vi "REPORT.Rate scan.vi"(9 "Vasic":i32, 10 "Config Test IN":T1={"Config HW"={"VISA Rigol DP832"="USB0::0x1AB1::0x0E11::DP8C191500901::INSTR", "Config Rigol DP832"=[{"Channel"=0, "V Limit"=5.5, "I Limit"=0.5, "V Out"=5.0}, {"Channel"=1, "V Limit"=5.5, "I Limit"=0.8, "V Out"=5.0}, {"Channel"=2, "V Limit"=5.5, "I Limit"=0.2, "V Out"=0.0}], "CTA Test#"="CTA013 A", "FT_Handle"=432866568, "Espera acceso FT"=10, "VISA Tek MDO3104"="Rigol_DP832", "VISA Key 81160A"="Rigol_DP832"}, "Config Test"=[{"Vasic"=2.8, "Global Reset"=FALSE, "Test Register?"=FALSE, "Test ADC?"=FALSE, "Test ADC"={"Repeats ADC"=100, "Max Desviation"=0.1}, "Limits ADC"={"Low"=[1.9, 1.3, 0.65, 0.0, 1.6, 1.4, 1.4, 0.9, 2.1, 0.85, 1.9], "High"=[2.1, 1.5, 0.85, 0.1, 1.4, 1.2, 1.2, 0.7, 1.9, 0.65, 1.7]}, "Test Max PN Min NP?"=FALSE, "Limits Max PN Min NP"={"Max P Upper"=2.177000045776367, "Min P Upper"=1.474, "Max N Upper"=1.475, "Min N Upper"=0.818, "Max P Lower"=1.888, "Min P Lower "=1.321, "Max N Lower"=1.322, "Min N Lower"=0.73}, "Test Rate Scan?"=FALSE, "Vin Rate Scan"=[], "Limits Rate Scan"={"High"=[0.15, 0.242, 0.331, 0.425, 0.512, 0.6, 0.688, 0.774, 0.847, 0.91], "Low"=[0.021, 0.11, 0.189, 0.27, 0.347, 0.421, 0.487, 0.551, 0.601, 0.635]}, "Test Rate Scan Adders?"=FALSE, "Vin Rate Adders"=[], "Limits Rate Scan adders"={"High"=[], "Low"=[]}, "Test offset analog?"=FALSE, "Lim Offset Analog"={"Max Analog"=0.05, "Min Analog"=-0.05}, "Test offset digital?"=FALSE, "Lim offset Dig"={"Max Dig"=0.05}, "Vasic real f.a."=2.8, "IBIAS"=FALSE, "VALUE IBIAS"=63}, {"Vasic"=2.8, "Global Reset"=FALSE, "Test Register?"=FALSE, "Test ADC?"=FALSE, "Test ADC"={"Repeats ADC"=100, "Max Desviation"=0.1}, "Limits ADC"={"Low"=[1.9, 1.3, 0.65, 0.0, 1.6, 1.4, 1.4, 0.9, 2.1, 0.85, 1.9], "High"=[2.1, 1.5, 0.85, 0.1, 1.4, 1.2, 1.2, 0.7, 1.9, 0.65, 1.7]}, "Test Max PN Min NP?"=FALSE, "Limits Max PN Min NP"={"Max P Upper"=2.177000045776367, "Min P Upper"=1.474, "Max N Upper"=1.475, "Min N Upper"=0.818, "Max P Lower"=1.888, "Min P Lower "=1.321, "Max N Lower"=1.322, "Min N Lower"=0.73}, "Test Rate Scan?"=FALSE, "Vin Rate Scan"=[], "Limits Rate Scan"={"High"=[0.15, 0.242, 0.331, 0.425, 0.512, 0.6, 0.688, 0.774, 0.847, 0.91], "Low"=[0.021, 0.11, 0.189, 0.27, 0.347, 0.421, 0.487, 0.551, 0.601, 0.635]}, "Test Rate Scan Adders?"=FALSE, "Vin Rate Adders"=[], "Limits Rate Scan adders"={"High"=[], "Low"=[]}, "Test offset analog?"=FALSE, "Lim Offset Analog"={"Max Analog"=0.05, "Min Analog"=-0.05}, "Test offset digital?"=FALSE, "Lim offset Dig"={"Max Dig"=0.05}, "Vasic real f.a."=2.8, "IBIAS"=FALSE, "VALUE IBIAS"=63}, {"Vasic"=2.8, "Global Reset"=FALSE, "Test Register?"=FALSE, "Test ADC?"=FALSE, "Test ADC"={"Repeats ADC"=100, "Max Desviation"=0.1}, "Limits ADC"={"Low"=[1.9, 1.3, 0.65, 0.0, 1.6, 1.4, 1.4, 0.9, 2.1, 0.85, 1.9], "High"=[2.1, 1.5, 0.85, 0.1, 1.4, 1.2, 1.2, 0.7, 1.9, 0.65, 1.7]}, "Test Max PN Min NP?"=FALSE, "Limits Max PN Min NP"={"Max P Upper"=2.177000045776367, "Min P Upper"=1.474, "Max N Upper"=1.475, "Min N Upper"=0.818, "Max P Lower"=1.888, "Min P Lower "=1.321, "Max N Lower"=1.322, "Min N Lower"=0.73}, "Test Rate Scan?"=FALSE, "Vin Rate Scan"=[], "Limits Rate Scan"={"High"=[0.15, 0.242, 0.331, 0.425, 0.512, 0.6, 0.688, 0.774, 0.847, 0.91], "Low"=[0.021, 0.11, 0.189, 0.27, 0.347, 0.421, 0.487, 0.551, 0.601, 0.635]}, "Test Rate Scan Adders?"=FALSE, "Vin Rate Adders"=[], "Limits Rate Scan adders"={"High"=[], "Low"=[]}, "Test offset analog?"=FALSE, "Lim Offset Analog"={"Max Analog"=0.05, "Min Analog"=-0.05}, "Test offset digital?"=FALSE, "Lim offset Dig"={"Max Dig"=0.05}, "Vasic real f.a."=2.8, "IBIAS"=FALSE, "VALUE IBIAS"=63}, {"Vasic"=2.8, "Global Reset"=FALSE, "Test Register?"=FALSE, "Test ADC?"=FALSE, "Test ADC"={"Repeats ADC"=100, "Max Desviation"=0.1}, "Limits ADC"={"Low"=[1.9, 1.3, 0.65, 0.0, 1.6, 1.4, 1.4, 0.9, 2.1, 0.85, 1.9], "High"=[2.1, 1.5, 0.85, 0.1, 1.4, 1.2, 1.2, 0.7, 1.9, 0.65, 1.7]}, "Test Max PN Min NP?"=FALSE, "Limits Max PN Min NP"={"Max P Upper"=2.177000045776367, "Min P Upper"=1.474, "Max N Upper"=1.475, "Min N Upper"=0.818, "Max P Lower"=1.888, "Min P Lower "=1.321, "Max N Lower"=1.322, "Min N Lower"=0.73}, "Test Rate Scan?"=FALSE, "Vin Rate Scan"=[], "Limits Rate Scan"={"High"=[0.15, 0.242, 0.331, 0.425, 0.512, 0.6, 0.688, 0.774, 0.847, 0.91], "Low"=[0.021, 0.11, 0.189, 0.27, 0.347, 0.421, 0.487, 0.551, 0.601, 0.635]}, "Test Rate Scan Adders?"=FALSE, "Vin Rate Adders"=[], "Limits Rate Scan adders"={"High"=[], "Low"=[]}, "Test offset analog?"=FALSE, "Lim Offset Analog"={"Max Analog"=0.05, "Min Analog"=-0.05}, "Test offset digital?"=FALSE, "Lim offset Dig"={"Max Dig"=0.05}, "Vasic real f.a."=2.8, "IBIAS"=FALSE, "VALUE IBIAS"=63}], "Result"=[{"Vasic Volt"=0, "Test Registros"={"Default Register OK"=FALSE, "Pattern Default"=[], "Read Default"=[], "W/R Register OK"=FALSE, "Pattern W/R"=[], "Read W/R"=[]}, "Test Dacs"={"Desviacion OK"=FALSE, "Means"=[], "Deviations"=[], "Desviations OK"=[], "Means OK"=[], "Graph Histogram"=[]}, "Test Max-Min PN"={"Max P Mini N OK"=FALSE, "PTHT Max P Min N"=[], "PTHT Max P Min N OK"=[], "NTHT Max P Min N"=[], "NTHT Max P Min N OK"=[], "Min P Max N OK"=FALSE, "PTHT Max N Min P"=[], "PTHT Max N Min P OK"=[], "NTHT Max N Min P"=[], "NTHT Max N Min P OK"=[], "Ref"=[]}, "Test Rate Scan"={"Rate Scan OK"=FALSE, "DAC TH0,TH1,TH2"=[], "Volt HLTH"=[], "Rate HLTH OK"=[], "DAC TH3,TH4,TH5"=[], "Volt LLTH"=[], "Rate LLTH 2 OK"=[], "Scaler 0"=[], "Ref"=[], "OFFSET HLTH"=[], "OFFSET LLTH"=[], "Real Voltage"=[]}, "Test Rate Scan adders"={"Rate Scan Adders OK"=FALSE, "DAC TH0,TH1,TH2"=[], "Volt HLTH"=[], "Add HLTH OK"=[], "DAC TH3,TH4,TH5"=[], "Volt LLTH"=[], "Add LLTH 2 OK"=[], "Scaler 0"=[], "Ref"=[], "OFFSET HLTH"=[], "OFFSET LLTH"=[], "Real Voltage"=[]}, "Test Offset Analog"={"Offset Analog OK"=FALSE, "V ADDOUT"=[], "Offset OK"=[], "Ref"=[]}, "Test Offset Digital"={"Offset Digital OK"=FALSE, "SCALER 1 START"=[], "SCALER 1 STOP"=[], "THX START"=[], "THX STOP"=[], "VHLTH START"=[], "VHLTH STOP"=[], "Index 1 Start"=[], "index 1 Stop"=[], "SCALER 2 START"=[], "SCALER 2 STOP"=[], "THX+3 START"=[], "THX+3 STOP"=[], "VLLTH START"=[], "VLLTH STOP"=[], "Index 2 Start"=[], "index 2 Stop"=[], "Dig HLTH OK"=[], "Dig LLTH 2 OK"=[], "Ref"=[]}, "info hardware"={"Iout V1"=0.0, "Iout V2"=0.0, "Iout V3"=0.0, "Vout V1"=0.0, "Vout V2"=0.0, "Vout V3"=0.0, "Temp"=0.0}, "Test Offset Analog add"={"Offset Analog add OK"=FALSE, "V ADDOUT add"=[], "Offset add OK"=[], "Ref add"=[]}, "info temp"={"T Asic Registers"=0.0, "T Board Test. ADC"=0.0, "T Asic Max Min N P"=0.0, "T Adc count"=0.0, "T Asic Digital Offset"=0.0, "T Asic Analog Offset"=0.0, "T Asic Analog add"=0.0, "T Asic Rate Scan"=0.0, "T Asic Rate Scan Adders"=0.0, "T Final"=0.0}}, {"Vasic Volt"=0, "Test Registros"={"Default Register OK"=FALSE, "Pattern Default"=[], "Read Default"=[], "W/R Register OK"=FALSE, "Pattern W/R"=[], "Read W/R"=[]}, "Test Dacs"={"Desviacion OK"=FALSE, "Means"=[], "Deviations"=[], "Desviations OK"=[], "Means OK"=[], "Graph Histogram"=[]}, "Test Max-Min PN"={"Max P Mini N OK"=FALSE, "PTHT Max P Min N"=[], "PTHT Max P Min N OK"=[], "NTHT Max P Min N"=[], "NTHT Max P Min N OK"=[], "Min P Max N OK"=FALSE, "PTHT Max N Min P"=[], "PTHT Max N Min P OK"=[], "NTHT Max N Min P"=[], "NTHT Max N Min P OK"=[], "Ref"=[]}, "Test Rate Scan"={"Rate Scan OK"=FALSE, "DAC TH0,TH1,TH2"=[], "Volt HLTH"=[], "Rate HLTH OK"=[], "DAC TH3,TH4,TH5"=[], "Volt LLTH"=[], "Rate LLTH 2 OK"=[], "Scaler 0"=[], "Ref"=[], "OFFSET HLTH"=[], "OFFSET LLTH"=[], "Real Voltage"=[]}, "Test Rate Scan adders"={"Rate Scan Adders OK"=FALSE, "DAC TH0,TH1,TH2"=[], "Volt HLTH"=[], "Add HLTH OK"=[], "DAC TH3,TH4,TH5"=[], "Volt LLTH"=[], "Add LLTH 2 OK"=[], "Scaler 0"=[], "Ref"=[], "OFFSET HLTH"=[], "OFFSET LLTH"=[], "Real Voltage"=[]}, "Test Offset Analog"={"Offset Analog OK"=FALSE, "V ADDOUT"=[], "Offset OK"=[], "Ref"=[]}, "Test Offset Digital"={"Offset Digital OK"=FALSE, "SCALER 1 START"=[], "SCALER 1 STOP"=[], "THX START"=[], "THX STOP"=[], "VHLTH START"=[], "VHLTH STOP"=[], "Index 1 Start"=[], "index 1 Stop"=[], "SCALER 2 START"=[], "SCALER 2 STOP"=[], "THX+3 START"=[], "THX+3 STOP"=[], "VLLTH START"=[], "VLLTH STOP"=[], "Index 2 Start"=[], "index 2 Stop"=[], "Dig HLTH OK"=[], "Dig LLTH 2 OK"=[], "Ref"=[]}, "info hardware"={"Iout V1"=0.0, "Iout V2"=0.0, "Iout V3"=0.0, "Vout V1"=0.0, "Vout V2"=0.0, "Vout V3"=0.0, "Temp"=0.0}, "Test Offset Analog add"={"Offset Analog add OK"=FALSE, "V ADDOUT add"=[], "Offset add OK"=[], "Ref add"=[]}, "info temp"={"T Asic Registers"=0.0, "T Board Test. ADC"=0.0, "T Asic Max Min N P"=0.0, "T Adc count"=0.0, "T Asic Digital Offset"=0.0, "T Asic Analog Offset"=0.0, "T Asic Analog add"=0.0, "T Asic Rate Scan"=0.0, "T Asic Rate Scan Adders"=0.0, "T Final"=0.0}}, {"Vasic Volt"=0, "Test Registros"={"Default Register OK"=FALSE, "Pattern Default"=[], "Read Default"=[], "W/R Register OK"=FALSE, "Pattern W/R"=[], "Read W/R"=[]}, "Test Dacs"={"Desviacion OK"=FALSE, "Means"=[], "Deviations"=[], "Desviations OK"=[], "Means OK"=[], "Graph Histogram"=[]}, "Test Max-Min PN"={"Max P Mini N OK"=FALSE, "PTHT Max P Min N"=[], "PTHT Max P Min N OK"=[], "NTHT Max P Min N"=[], "NTHT Max P Min N OK"=[], "Min P Max N OK"=FALSE, "PTHT Max N Min P"=[], "PTHT Max N Min P OK"=[], "NTHT Max N Min P"=[], "NTHT Max N Min P OK"=[], "Ref"=[]}, "Test Rate Scan"={"Rate Scan OK"=FALSE, "DAC TH0,TH1,TH2"=[], "Volt HLTH"=[], "Rate HLTH OK"=[], "DAC TH3,TH4,TH5"=[], "Volt LLTH"=[], "Rate LLTH 2 OK"=[], "Scaler 0"=[], "Ref"=[], "OFFSET HLTH"=[], "OFFSET LLTH"=[], "Real Voltage"=[]}, "Test Rate Scan adders"={"Rate Scan Adders OK"=FALSE, "DAC TH0,TH1,TH2"=[], "Volt HLTH"=[], "Add HLTH OK"=[], "DAC TH3,TH4,TH5"=[], "Volt LLTH"=[], "Add LLTH 2 OK"=[], "Scaler 0"=[], "Ref"=[], "OFFSET HLTH"=[], "OFFSET LLTH"=[], "Real Voltage"=[]}, "Test Offset Analog"={"Offset Analog OK"=FALSE, "V ADDOUT"=[], "Offset OK"=[], "Ref"=[]}, "Test Offset Digital"={"Offset Digital OK"=FALSE, "SCALER 1 START"=[], "SCALER 1 STOP"=[], "THX START"=[], "THX STOP"=[], "VHLTH START"=[], "VHLTH STOP"=[], "Index 1 Start"=[], "index 1 Stop"=[], "SCALER 2 START"=[], "SCALER 2 STOP"=[], "THX+3 START"=[], "THX+3 STOP"=[], "VLLTH START"=[], "VLLTH STOP"=[], "Index 2 Start"=[], "index 2 Stop"=[], "Dig HLTH OK"=[], "Dig LLTH 2 OK"=[], "Ref"=[]}, "info hardware"={"Iout V1"=0.0, "Iout V2"=0.0, "Iout V3"=0.0, "Vout V1"=0.0, "Vout V2"=0.0, "Vout V3"=0.0, "Temp"=0.0}, "Test Offset Analog add"={"Offset Analog add OK"=FALSE, "V ADDOUT add"=[], "Offset add OK"=[], "Ref add"=[]}, "info temp"={"T Asic Registers"=0.0, "T Board Test. ADC"=0.0, "T Asic Max Min N P"=0.0, "T Adc count"=0.0, "T Asic Digital Offset"=0.0, "T Asic Analog Offset"=0.0, "T Asic Analog add"=0.0, "T Asic Rate Scan"=0.0, "T Asic Rate Scan Adders"=0.0, "T Final"=0.0}}, {"Vasic Volt"=0, "Test Registros"={"Default Register OK"=FALSE, "Pattern Default"=[], "Read Default"=[], "W/R Register OK"=FALSE, "Pattern W/R"=[], "Read W/R"=[]}, "Test Dacs"={"Desviacion OK"=FALSE, "Means"=[], "Deviations"=[], "Desviations OK"=[], "Means OK"=[], "Graph Histogram"=[]}, "Test Max-Min PN"={"Max P Mini N OK"=FALSE, "PTHT Max P Min N"=[], "PTHT Max P Min N OK"=[], "NTHT Max P Min N"=[], "NTHT Max P Min N OK"=[], "Min P Max N OK"=FALSE, "PTHT Max N Min P"=[], "PTHT Max N Min P OK"=[], "NTHT Max N Min P"=[], "NTHT Max N Min P OK"=[], "Ref"=[]}, "Test Rate Scan"={"Rate Scan OK"=FALSE, "DAC TH0,TH1,TH2"=[], "Volt HLTH"=[], "Rate HLTH OK"=[], "DAC TH3,TH4,TH5"=[], "Volt LLTH"=[], "Rate LLTH 2 OK"=[], "Scaler 0"=[], "Ref"=[], "OFFSET HLTH"=[], "OFFSET LLTH"=[], "Real Voltage"=[]}, "Test Rate Scan adders"={"Rate Scan Adders OK"=FALSE, "DAC TH0,TH1,TH2"=[], "Volt HLTH"=[], "Add HLTH OK"=[], "DAC TH3,TH4,TH5"=[], "Volt LLTH"=[], "Add LLTH 2 OK"=[], "Scaler 0"=[], "Ref"=[], "OFFSET HLTH"=[], "OFFSET LLTH"=[], "Real Voltage"=[]}, "Test Offset Analog"={"Offset Analog OK"=FALSE, "V ADDOUT"=[], "Offset OK"=[], "Ref"=[]}, "Test Offset Digital"={"Offset Digital OK"=FALSE, "SCALER 1 START"=[], "SCALER 1 STOP"=[], "THX START"=[], "THX STOP"=[], "VHLTH START"=[], "VHLTH STOP"=[], "Index 1 Start"=[], "index 1 Stop"=[], "SCALER 2 START"=[], "SCALER 2 STOP"=[], "THX+3 START"=[], "THX+3 STOP"=[], "VLLTH START"=[], "VLLTH STOP"=[], "Index 2 Start"=[], "index 2 Stop"=[], "Dig HLTH OK"=[], "Dig LLTH 2 OK"=[], "Ref"=[]}, "info hardware"={"Iout V1"=0.0, "Iout V2"=0.0, "Iout V3"=0.0, "Vout V1"=0.0, "Vout V2"=0.0, "Vout V3"=0.0, "Temp"=0.0}, "Test Offset Analog add"={"Offset Analog add OK"=FALSE, "V ADDOUT add"=[], "Offset add OK"=[], "Ref add"=[]}, "info temp"={"T Asic Registers"=0.0, "T Board Test. ADC"=0.0, "T Asic Max Min N P"=0.0, "T Adc count"=0.0, "T Asic Digital Offset"=0.0, "T Asic Analog Offset"=0.0, "T Asic Analog add"=0.0, "T Asic Rate Scan"=0.0, "T Asic Rate Scan Adders"=0.0, "T Final"=0.0}}], "Execucion Test"={"Vasic Actual"=0}, "Config VGA"={"Theoretical Voltage"=[0.1, 0.2, 0.3, 0.4, 0.5, 0.6, 0.7, 0.8, 0.9, 1.0], "Real Voltage"=[0.10285, 0.20714, 0.29957, 0.40485, 0.49571, 0.60685, 0.69771, 0.80114, 0.89714, 0.99885], "Pulse Width"=57344, "Frecuency Pulse"=1000000.0, "VGA Gain"=[9, 16, 24, 34, 43, 52, 61, 72, 81, 93]}, "Test Info"={"Asic"="", "Operator"="", "Place"="", "Time start"=timestamp(0 s since 1904-01-01), "Time stop"=timestamp(0 s since 1904-01-01)}, "Info machine"={"SO"="", "SO Name"="", "SO Ver"="", "SO Build"="", "CPU"="", "APP"="", "APP YEAR"="", "APP ver"="", "APP User"="", "APP Serail"="", "MAC"=[], "PC NAME"=[], "PC IP"=[], "BIOS MANU"="", "BIOS NAME"="", "BIOS SERIAL"="", "BOARD MANU"="", "BOARD NAME"="", "BOARD SERIAL"="", "Driver Version"="", "Library Version"="", "FPGA Ver"=0, "ID CTA board"=0, "LAST BOOT"="", "LABVIEW Ver"=0}, "Partial Report"="", "CONFIG GEN"=[]} {"CONFIG GEN"."Vasic Theorical" min=1.0 max=1000000.0 step=1.0 format="%#_6pV"; "CONFIG GEN"."Frequency" min=0.001 max=333000000.0 step=1000.0 format="%#_6pHz"; "CONFIG GEN"."Leading Edge Time" min=1e-09 max=1.0 step=1e-10 format="%#_6ps"; "CONFIG GEN"."Trailing Edge Time" min=1e-09 max=1.0 step=1e-10 format="%#_6ps"; "CONFIG GEN"."Delay" min=0.0 max=1.0 step=1e-12 format="%#_6ps"; "CONFIG GEN"."Trigger Level Sync" items=["ECL", "TTL"]; "CONFIG GEN"."Trigger Sync Out" items=["AB"=3, "B"=2, "A"=1, "None"=0]; "CONFIG GEN"."Load" min=1.0 max=1000000.0 step=1.0 format="%#_6p"; "CONFIG GEN"."DC Offset" min=-10.0 max=10.0 step=0.1 format="%#_6pV"; "CONFIG GEN"."Amplitude" min=0.05 max=5.0 step=0.001 format="%#_6pV"; "CONFIG GEN"."Width Time" min=1.5e-09 max=1.0 step=1e-10 format="%#_6ps"; "CONFIG GEN"."Channel" items=["Channel1"=1, "Channel2"=2]; "Config VGA"."Theoretical Voltage" format="%1.4f"; "Config VGA"."VGA Gain" format="%02x"; "Config VGA"."Frecuency Pulse" format="%0_2p"; "Config VGA"."Pulse Width" format="%04x"; "Config VGA"."Real Voltage" format="%1.5f"; "Config Test"."VALUE IBIAS" max=63 step=1; "Config Test"."Vasic real f.a." min=2.8 max=3.8 step=0.01 format="%.2g"; "Config Test"."Limits Rate Scan adders"."Low" format="%1.3f"; "Config Test"."Limits Rate Scan adders"."High" format="%1.3f"; "Config Test"."Limits ADC"."High" format="%1.4f"; "Config Test"."Limits ADC"."Low" format="%1.3f"; "Config Test"."Lim offset Dig"."Max Dig" format="%.3g"; "Config Test"."Lim Offset Analog"."Min Analog" format="%.3g"; "Config Test"."Lim Offset Analog"."Max Analog" format="%.3g"; "Config Test"."Limits Rate Scan"."Low" format="%1.4f"; "Config Test"."Limits Rate Scan"."High" format="%1.3f"; "Config Test"."Limits Max PN Min NP"."Min P Upper" format="%.3g"; "Config Test"."Limits Max PN Min NP"."Min P Lower" format="%.3g"; "Config Test"."Limits Max PN Min NP"."Max N Lower" format="%.3g"; "Config Test"."Limits Max PN Min NP"."Max N Upper" format="%.3g"; "Config Test"."Limits Max PN Min NP"."Min N Lower" format="%.3g"; "Config Test"."Limits Max PN Min NP"."Min N Upper" format="%.3g"; "Config Test"."Limits Max PN Min NP"."Max P Upper" format="%.3g"; "Config Test"."Limits Max PN Min NP"."Max P Lower" format="%.3g"; "Config Test"."Vasic" min=2.8 max=3.8 step=0.01 format="%.2g"; "Config HW"."Config Rigol DP832"."Channel" items=["+30V Channel 1", "+30V Channel 2", "+5V Channel 3"]; "Config HW"."Config Rigol DP832"."V Limit" format="%.1g"; "Config HW"."Config Rigol DP832"."I Limit" format="%.1g"; "Config HW"."Config Rigol DP832"."V Out" format="%.1g"; "Result"."Test Registros"."Read W/R" format="%04x"; "Result"."Test Registros"."Pattern W/R" format="%04x"; "Result"."Test Registros"."Read Default" format="%04x"; "Result"."Test Registros"."Pattern Default" format="%04x"}, 11 "Text In":string) -> (3 "Text Out":string)   [LabVIEW 2019]
uses:
  Test.ctl
  TEST.TEST CONFIG HW.ctl
  Rigol DP832/DP832_Control Channels.ctl
  TEST.TEST CONFIG TEST MATRIZ.ctl
  TEST.TEST CONFIG TEST.ctl
  TEST.TEST RESULT.ctl
  test_result fvasic.ctl
  TEST.TEST EXECUTION TEST.ctl
  TEST.TEST CONFIG VGA.ctl
  TEST.TEST TEST INFO.ctl
  TEST.TEST INFO PC.ctl
  GenPulse_configurar.ctl
panel:
  out "Test Rate Scan.OFFSET LLTH":dbl[][](array[numeric])
  out "Test Rate Scan.OFFSET HLTH":dbl[][](array[numeric])
  out "Salida B rectificada":dbl[][][](array[numeric])
  out "Salida A rectificada":dbl[][][](array[numeric])
  # "Modo 2\nModo 3\nModo 4\nModo 2\nModo 3\nModo 4"
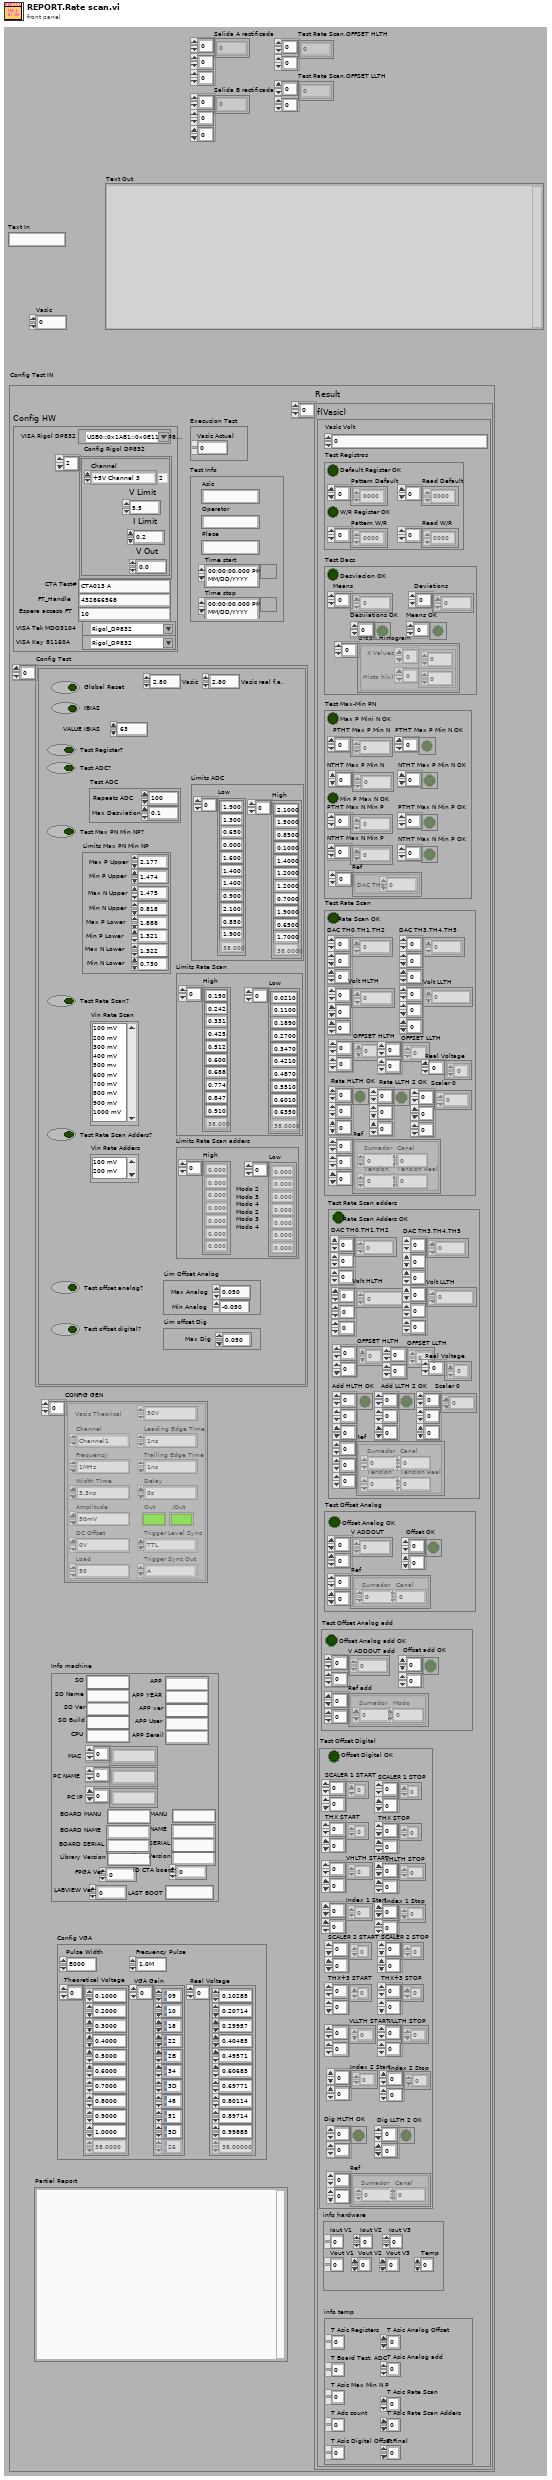
[diagram p1: front panel]
types:
  T1 = typedef "Test.ctl" = cluster{"Config HW":T2, "Config Test":T4, "Result":T6, "Execucion Test":T8, "Config VGA":T9, "Test Info":T10, "Info machine":T11, "Partial Report":string, "CONFIG GEN":T12[]}
  T2 = typedef "TEST.TEST CONFIG HW.ctl" = cluster{"VISA Rigol DP832":refnum<visa-resource-name>, "Config Rigol DP832":cluster{"Channel":T3, "V Limit":dbl, "I Limit":dbl, "V Out":dbl}[], "CTA Test#":string, "FT_Handle":u32, "Espera acceso FT":u32, "VISA Tek MDO3104":refnum<visa-resource-name>, "VISA Key 81160A":refnum<visa-resource-name>}
  T3 = typedef "DP832_Control Channels.ctl" = i32
  T4 = typedef "TEST.TEST CONFIG TEST MATRIZ.ctl" = T5[]
  T5 = typedef "TEST.TEST CONFIG TEST.ctl" = cluster{"Vasic":dbl, "Global Reset":bool, "Test Register?":bool, "Test ADC?":bool, "Test ADC":cluster{"Repeats ADC":i32, "Max Desviation":dbl}, "Limits ADC":cluster{"Low":dbl[], "High":dbl[]}, "Test Max PN Min NP?":bool, "Limits Max PN Min NP":cluster{"Max P Upper":dbl, "Min P Upper":dbl, "Max N Upper":dbl, "Min N Upper":dbl, "Max P Lower":dbl, "Min P Lower ":dbl, "Max N Lower":dbl, "Min N Lower":dbl}, "Test Rate Scan?":bool, "Vin Rate Scan":i32[], "Limits Rate Scan":cluster{"High":dbl[], "Low":dbl[]}, "Test Rate Scan Adders?":bool, "Vin Rate Adders":i32[], "Limits Rate Scan adders":cluster{"High":dbl[], "Low":dbl[]}, "Test offset analog?":bool, "Lim Offset Analog":cluster{"Max Analog":dbl, "Min Analog":dbl}, "Test offset digital?":bool, "Lim offset Dig":cluster{"Max Dig":dbl}, "Vasic real f.a.":dbl, "IBIAS":bool, "VALUE IBIAS":u8}
  T6 = typedef "TEST.TEST RESULT.ctl" = T7[]
  T7 = typedef "test_result fvasic.ctl" = cluster{"Vasic Volt":i32, "Test Registros":cluster{"Default Register OK":bool, "Pattern Default":u16[], "Read Default":u16[], "W/R Register OK":bool, "Pattern W/R":u16[], "Read W/R":u16[]}, "Test Dacs":cluster{"Desviacion OK":bool, "Means":dbl[], "Deviations":dbl[], "Desviations OK":bool[], "Means OK":bool[], "Graph Histogram":cluster{"X Values":dbl[], "Histo h(x)":i32[]}[]}, "Test Max-Min PN":cluster{"Max P Mini N OK":bool, "PTHT Max P Min N":dbl[], "PTHT Max P Min N OK":bool[], "NTHT Max P Min N":dbl[], "NTHT Max P Min N OK":bool[], "Min P Max N OK":bool, "PTHT Max N Min P":dbl[], "PTHT Max N Min P OK":bool[], "NTHT Max N Min P":dbl[], "NTHT Max N Min P OK":bool[], "Ref":cluster{"DAC THx":u8}[]}, "Test Rate Scan":cluster{"Rate Scan OK":bool, "DAC TH0,TH1,TH2":u16[][][], "Volt HLTH":dbl[][][], "Rate HLTH OK":bool[][][], "DAC TH3,TH4,TH5":u16[][][], "Volt LLTH":dbl[][][], "Rate LLTH 2 OK":bool[][][], "Scaler 0":u16[][][], "Ref":cluster{"Sumador":u8, "Canal":u8, "Tension":u8, "Tension Real":dbl}[][][], "OFFSET HLTH":dbl[][], "OFFSET LLTH":dbl[][], "Real Voltage":dbl[]}, "Test Rate Scan adders":cluster{"Rate Scan Adders OK":bool, "DAC TH0,TH1,TH2":u16[][][], "Volt HLTH":dbl[][][], "Add HLTH OK":bool[][][], "DAC TH3,TH4,TH5":u16[][][], "Volt LLTH":dbl[][][], "Add LLTH 2 OK":bool[][][], "Scaler 0":u16[][][], "Ref":cluster{"Sumador":u8, "Canal":u8, "Tension":u8, "Tension Real":dbl}[][][], "OFFSET HLTH":dbl[][], "OFFSET LLTH":dbl[][], "Real Voltage":dbl[]}, "Test Offset Analog":cluster{"Offset Analog OK":bool, "V ADDOUT":dbl[][], "Offset OK":bool[][], "Ref":cluster{"Sumador":u8, "Canal":u8}[][]}, "Test Offset Digital":cluster{"Offset Digital OK":bool, "SCALER 1 START":u16[][], "SCALER 1 STOP":u16[][], "THX START":u16[][], "THX STOP":u16[][], "VHLTH START":dbl[][], "VHLTH STOP":dbl[][], "Index 1 Start":i32[][], "index 1 Stop":i32[][], "SCALER 2 START":u16[][], "SCALER 2 STOP":u16[][], "THX+3 START":u16[][], "THX+3 STOP":u16[][], "VLLTH START":dbl[][], "VLLTH STOP":dbl[][], "Index 2 Start":i32[][], "index 2 Stop":i32[][], "Dig HLTH OK":bool[][], "Dig LLTH 2 OK":bool[][], "Ref":cluster{"Sumador":u8, "Canal":u8}[][]}, "info hardware":cluster{"Iout V1":dbl, "Iout V2":dbl, "Iout V3":dbl, "Vout V1":dbl, "Vout V2":dbl, "Vout V3":dbl, "Temp":dbl}, "Test Offset Analog add":cluster{"Offset Analog add OK":bool, "V ADDOUT add":dbl[][], "Offset add OK":bool[][], "Ref add":cluster{"Sumador":u8, "Modo":u8}[][]}, "info temp":cluster{"T Asic Registers":dbl, "T Board Test. ADC":dbl, "T Asic Max Min N P":dbl, "T Adc count":dbl, "T Asic Digital Offset":dbl, "T Asic Analog Offset":dbl, "T Asic Analog add":dbl, "T Asic Rate Scan":dbl, "T Asic Rate Scan Adders":dbl, "T Final":dbl}}
  T8 = typedef "TEST.TEST EXECUTION TEST.ctl" = cluster{"Vasic Actual":i32}
  T9 = typedef "TEST.TEST CONFIG VGA.ctl" = cluster{"Theoretical Voltage":dbl[], "Real Voltage":dbl[], "Pulse Width":u16, "Frecuency Pulse":dbl, "VGA Gain":u8[]}
  T10 = typedef "TEST.TEST TEST INFO.ctl" = cluster{"Asic":string, "Operator":string, "Place":string, "Time start":timestamp, "Time stop":timestamp}
  T11 = typedef "TEST.TEST INFO PC.ctl" = cluster{"SO":string, "SO Name":string, "SO Ver":string, "SO Build":string, "CPU":string, "APP":string, "APP YEAR":string, "APP ver":string, "APP User":string, "APP Serail":string, "MAC":string[], "PC NAME":string[], "PC IP":string[], "BIOS MANU":string, "BIOS NAME":string, "BIOS SERIAL":string, "BOARD MANU":string, "BOARD NAME":string, "BOARD SERIAL":string, "Driver Version":string, "Library Version":string, "FPGA Ver":u8, "ID CTA board":u64, "LAST BOOT":string, "LABVIEW Ver":u32}
  T12 = typedef "GenPulse_configurar.ctl" = cluster{"Channel":u16, "Frequency":dbl, "Width Time":dbl, "Amplitude":dbl, "DC Offset":dbl, "Load":dbl, "Leading Edge Time":dbl, "Trailing Edge Time":dbl, "Delay":dbl, "Out":bool, "/Out":bool, "Trigger Level Sync":u16, "Trigger Sync Out":u16, "Vasic Theorical":dbl}
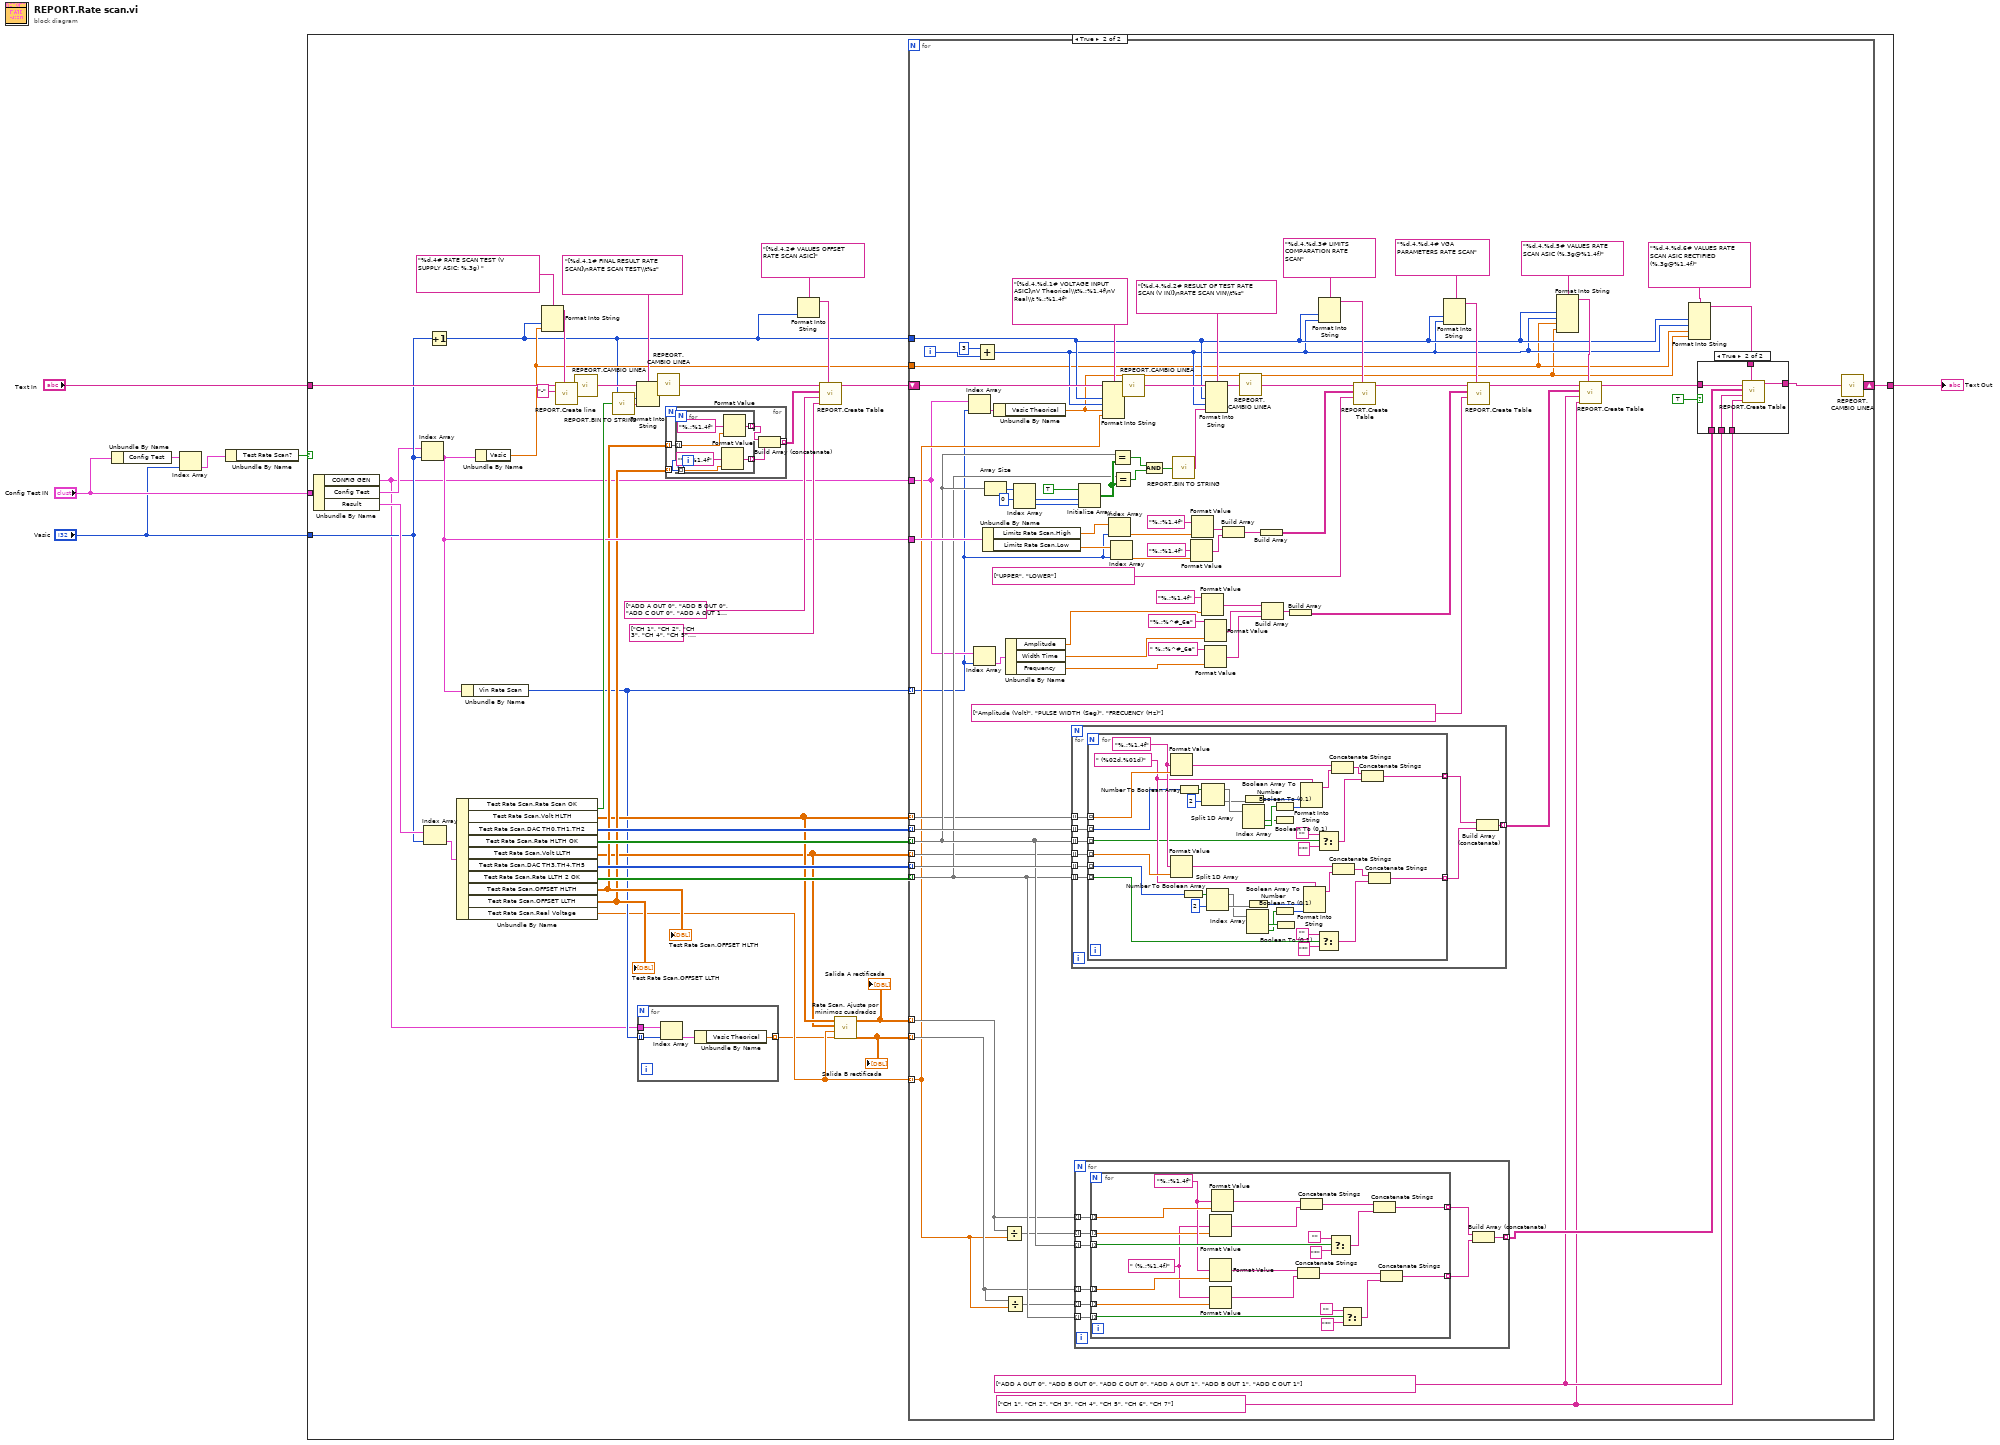
[diagram p0: block diagram]
diagram:
  n1 = Unbundle By Name("Config Test IN") -> ("Config Test"=w5:T4)
  n2 = Index Array(array=w5, index="Vasic") -> (element=w4:T5)
  n3 = Unbundle By Name(w4) -> ("Test Rate Scan?"=w2:bool)
  n4 = case shown="True" w2 {
    tunnel: "Text In" -> [w8 w48]
    tunnel: [w8 w44] -> w6
    tunnel: "Vasic" -> [_ w37]
    tunnel: "Config Test IN" -> [_ w30]
    frame False {
    }
    frame True {
      n5 = Unbundle By Name(w30) -> ("CONFIG GEN"=w9:T12[], "Config Test"=w13:T4, "Result"=w42:T6)
      n6 = Index Array(array=w13, index=w37) -> (element=w21:T5)
      n7 = Index Array(array=w42, index=w37) -> (element=w47:T7)
      n8 = Increment(x=w37) -> (x+1=w24:i32)
      n9 = Unbundle By Name(w47) -> ("Test Rate Scan.Rate Scan OK"=w32:bool, "Test Rate Scan.Volt HLTH"=w17:dbl[][][], "Test Rate Scan.DAC TH0,TH1,TH2"=w46:u16[][][], "Test Rate Scan.Rate HLTH OK"=w41:bool[][][], "Test Rate Scan.Volt LLTH"=w16:dbl[][][], "Test Rate Scan.DAC TH3,TH4,TH5"=w45:u16[][][], "Test Rate Scan.Rate LLTH 2 OK"=w40:bool[][][], "Test Rate Scan.OFFSET HLTH"=w20:dbl[][], "Test Rate Scan.OFFSET LLTH"=w19:dbl[][], "Test Rate Scan.Real Voltage"=w11:dbl[])
      "Test Rate Scan.OFFSET HLTH" <- w20
      "Test Rate Scan.OFFSET LLTH" <- w19
      n10 = Unbundle By Name(w21) -> ("Vin Rate Scan"=w12:i32[])
      n11 = Unbundle By Name(w21) -> ("Vasic"=w25:dbl)
      n12 = Format Into String(format string="%d.4# RATE SCAN TEST (V SUPPLY ASIC: %.3g) " ("Secction"), w24, w25) -> (resulting string=w36:string)  [unwired: 2 in, 1 out]
      n13 = call "REPORT.Create line.vi"("Secction"=w36, "Char"="-", "Text In"=w48) -> ("Text Out"=w43:string)  [unwired: 8 in]
      n14 = call "REPEORT.CAMBIO LINEA.vi"("Text Out"=w43) -> ("String"=w34:string)  [unwired: 8 in]
      n15 = call "REPORT.BIN TO STRING.vi"("Resultado test"=w32) -> ("OK, Fault"=w33:string)  [unwired: 14 in]
      n16 = Format Into String(format string="[%d.4.1# FINAL RESULT RATE SCAN]\nRATE SCAN TEST\\t%s" ("Secction"), initial string=w34, w24, w33) -> (resulting string=w31:string)  [unwired: 1 in, 1 out]
      n17 = for {
        tunnel: w12 -> [w52] mode=indexing
        tunnel: w9 -> [w51]
        tunnel: [w49] -> w10 mode=indexing
        n18 = Index Array(array=w51, index=w52) -> (element=w50:T12)
        n19 = Unbundle By Name(w50) -> ("Vasic Theorical"=w49:dbl)
      }
      n20 = call "REPEORT.CAMBIO LINEA.vi"("Text Out"=w31) -> ("String"=w27:string)  [unwired: 8 in]
      n21 = for {
        tunnel: w20 -> [w57] mode=indexing
        tunnel: w19 -> [w56] mode=indexing
        tunnel: [w53] -> w18 mode=indexing
        n22 = for {
          tunnel: w57 -> [w61] mode=indexing
          tunnel: w56 -> [w60] mode=indexing
          tunnel: [w59] -> w55 mode=indexing
          tunnel: [w58] -> w54 mode=indexing
          n23 = Format Value(format string="%,;%1.4f", value (0)=w60) -> (output string=w58:string)  [unwired: 1 in]
          n24 = Format Value(format string="%,;%1.4f", value (0)=w61) -> (output string=w59:string)  [unwired: 1 in]
        }
        n25 = Build Array (concatenate)(w55, w54) -> (w53:string[])
      }
      n26 = Format Into String(format string="[%d.4.2# VALUES OFFSET RATE SCAN ASIC]" ("Secction"), w24) -> (resulting string=w29:string)  [unwired: 2 in, 1 out]
      n27 = call "REPORT.Create Table.vi"("Secction"=w29, "Row Headers"=string[] ["CH 1", "CH 2", "CH 3", "CH 4", "CH 5", "CH 6", "CH 7"], "Column Headers"=string[] ["ADD A OUT 0", "ADD B OUT 0", "ADD C OUT 0", "ADD A OUT 1", "ADD B OUT 1", "ADD C OUT 1"], "Text 2d"=w18, "Text In"=w27) -> ("Text Out"=w26:string)  [unwired: 3 in, 1 out]
      n28 = call "Rate Scan. Ajuste por minimos cuadrados.vi"("V asic Theorical"=w10, "V asic Real"=w11, "Salida B"=w16, "Salida A"=w17) -> ("Salida B rectificada"=w14:dbl[][][], "Salida A rectificada"=w15:dbl[][][])  [unwired: 2 out]
      "Salida A rectificada" <- w15
      "Salida B rectificada" <- w14
      n29 = for {
        tunnel: w17 -> [w82] mode=indexing
        tunnel: w46 -> [w143] mode=indexing
        tunnel: w16 -> [w81] mode=indexing
        tunnel: w45 -> [w142] mode=indexing
        shift-right: [w105] -> w44
        shift-left: w26 -> [w119]
        tunnel: w9 -> [w68]
        tunnel: w12 -> [w66] mode=indexing
        tunnel: w21 -> [w131]
        tunnel: w41 -> [w87] mode=indexing
        tunnel: w40 -> [w86] mode=indexing
        tunnel: w24 -> [w77]
        tunnel: w25 -> [w75]
        tunnel: w15 -> [w73] mode=indexing
        tunnel: w14 -> [w72] mode=indexing
        tunnel: w11 -> [w70] mode=indexing
        i -> [w103]
        w78 = string[] ["CH 1", "CH 2", "CH 3", "CH 4", "CH 5", "CH 6", "CH 7"] ("Row Headers")
        w79 = string[] ["ADD A OUT 0", "ADD B OUT 0", "ADD C OUT 0", "ADD A OUT 1", "ADD B OUT 1", "ADD C OUT 1"] ("Column Headers")
        n30 = Index Array(array=w68, index=w66) -> (element=w69:T12)
        n31 = Index Array(array=w68, index=w66) -> (element=w67:T12)
        n32 = Add(x=3, y=w103) -> (x+y=w76:i32)
        n33 = Unbundle By Name(w131) -> ("Limits Rate Scan.High"=w128:dbl[], "Limits Rate Scan.Low"=w127:dbl[])
        n34 = Array Size(array=w87) -> (size(s)=w113:i32[])
        n35 = Unbundle By Name(w69) -> ("Vasic Theorical"=w64:dbl)
        n36 = Divide(x=w73, y=w70) -> (x/y=w85:dbl[][])
        n37 = Divide(x=w72, y=w70) -> (x/y=w84:dbl[][])
        n38 = Unbundle By Name(w67) -> ("Amplitude"=w65:dbl, "Width Time"=w106:dbl, "Frequency"=w140:dbl)
        n39 = Index Array(array=w113, index #1=0 ("index")) -> (element #1=w111:i32, element #2=w110:i32)  [unwired: 1 in]
        n40 = for {
          tunnel: w82 -> [w190] mode=indexing
          tunnel: w143 -> [w189] mode=indexing
          tunnel: w81 -> [w188] mode=indexing
          tunnel: w142 -> [w187] mode=indexing
          tunnel: [w184] -> w89 mode=indexing
          tunnel: w87 -> [w183] mode=indexing
          tunnel: w86 -> [w182] mode=indexing
          n41 = for {
            tunnel: w190 -> [w228] mode=indexing
            tunnel: w189 -> [w193] mode=indexing
            tunnel: w188 -> [w227] mode=indexing
            tunnel: w187 -> [w205] mode=indexing
            tunnel: [w219] -> w186 mode=indexing
            tunnel: [w214] -> w185 mode=indexing
            tunnel: w183 -> [w192] mode=indexing
            tunnel: w182 -> [w191] mode=indexing
            w194 = " (%02d.%01d)" ("format string")
            w225 = "%,;%1.4f" ("format string")
            n42 = Format Value(format string=w225, value (0)=w228) -> (output string=w226:string)  [unwired: 1 in]
            n43 = Format Value(format string=w225, value (0)=w227) -> (output string=w224:string)  [unwired: 1 in]
            n44 = Number To Boolean Array(number=w193) -> (Boolean array=w196:bool[])
            n45 = Number To Boolean Array(number=w205) -> (Boolean array=w213:bool[])
            n46 = Split 1D Array(array=w196, index=2) -> (first subarray=w200:bool[], second subarray=w199:bool[])
            n47 = Split 1D Array(array=w213, index=2) -> (first subarray=w209:bool[], second subarray=w210:bool[])
            n48 = Index Array(array=w200) -> (element #1=w201:bool, element #2=w203:bool)  [unwired: 2 in]
            n49 = Boolean Array To Number(Boolean array=w199) -> (number=w198:u32)
            n50 = Index Array(array=w209) -> (element #1=w208:bool, element #2=w206:bool)  [unwired: 2 in]
            n51 = Boolean Array To Number(Boolean array=w210) -> (number=w211:u32)
            n52 = Boolean To (0,1)(Boolean=w203) -> (0, 1=w202:i16)
            n53 = Boolean To (0,1)(Boolean=w201) -> ()  [unwired: 1 out]
            n54 = Boolean To (0,1)(Boolean=w206) -> (0, 1=w207:i16)
            n55 = Boolean To (0,1)(Boolean=w208) -> ()  [unwired: 1 out]
            n56 = Format Into String(format string=w194, w198, w202) -> (resulting string=w195:string)  [unwired: 2 in, 1 out]
            n57 = Format Into String(format string=w194, w211, w207) -> (resulting string=w204:string)  [unwired: 2 in, 1 out]
            n58 = Select(t="", s=w192, f="*") -> (s? t:f=w221:string)
            n59 = Select(t="", s=w191, f="*") -> (s? t:f=w215:string)
            n60 = Concatenate Strings(w226, w195) -> (w220:string)
            n61 = Concatenate Strings(w224, w204) -> (w216:string)
            n62 = Concatenate Strings(w220, w221) -> (w219:string)
            n63 = Concatenate Strings(w216, w215) -> (w214:string)
          }
          n64 = Build Array (concatenate)(w186, w185) -> (w184:string[])
        }
        n65 = for {
          tunnel: w87 -> [w152] mode=indexing
          tunnel: w86 -> [w151] mode=indexing
          tunnel: w73 -> [w150] mode=indexing
          tunnel: w72 -> [w149] mode=indexing
          tunnel: w85 -> [w148] mode=indexing
          tunnel: w84 -> [w147] mode=indexing
          tunnel: [w144] -> w83 mode=indexing
          n66 = for {
            tunnel: w152 -> [w164] mode=indexing
            tunnel: w151 -> [w162] mode=indexing
            tunnel: w150 -> [w165] mode=indexing
            tunnel: w149 -> [w163] mode=indexing
            tunnel: w148 -> [w157] mode=indexing
            tunnel: w147 -> [w155] mode=indexing
            tunnel: [w161] -> w146 mode=indexing
            tunnel: [w160] -> w145 mode=indexing
            w153 = " (%,;%1.4f)" ("format string")
            w158 = "%,;%1.4f" ("format string")
            n67 = Format Value(format string=w153, value (0)=w157) -> (output string=w156:string)  [unwired: 1 in]
            n68 = Format Value(format string=w158, value (0)=w163) -> (output string=w166:string)  [unwired: 1 in]
            n69 = Format Value(format string=w153, value (0)=w155) -> (output string=w154:string)  [unwired: 1 in]
            n70 = Format Value(format string=w158, value (0)=w165) -> (output string=w159:string)  [unwired: 1 in]
            n71 = Concatenate Strings(w166, w154) -> (w173:string)
            n72 = Concatenate Strings(w159, w156) -> (w170:string)
            n73 = Select(t="", s=w164, f="*") -> (s? t:f=w169:string)
            n74 = Select(t="", s=w162, f="*") -> (s? t:f=w174:string)
            n75 = Concatenate Strings(w170, w169) -> (w161:string)
            n76 = Concatenate Strings(w173, w174) -> (w160:string)
          }
          n77 = Build Array (concatenate)(w146, w145) -> (w144:string[])
        }
        n78 = Initialize Array(TRUE, w111, w110) -> (w116:bool[][])
        n79 = Format Into String(format string="[%d.4.%d.1# VOLTAGE INPUT ASIC]\nV Theorical\\t%,;%1.4f\nV Real\\t %,;%1.4f" ("Secction"), initial string=w119, w77, w76, w64, w70) -> (resulting string=w102:string)  [unwired: 1 in, 1 out]
        n80 = Index Array(array=w128, index=w66) -> (element=w126:dbl)
        n81 = Index Array(array=w127, index=w66) -> (element=w125:dbl)
        n82 = Equal?(x=w87, y=w116) -> (x = y?=w115:bool)
        n83 = Equal?(x=w86, y=w116) -> (x = y?=w114:bool)
        n84 = call "REPEORT.CAMBIO LINEA.vi"("Text Out"=w102) -> ("String"=w101:string)  [unwired: 8 in]
        n85 = And(x=w115, y=w114) -> (x .and. y?=w109:bool)
        n86 = call "REPORT.BIN TO STRING.vi"("Resultado test"=w109) -> ("OK, Fault"=w92:string)  [unwired: 14 in]
        n87 = Format Value(format string="%,;%1.4f", value (0)=w125) -> (output string=w123:string)  [unwired: 1 in]
        n88 = Format Value(format string="%,;%1.4f", value (0)=w126) -> (output string=w124:string)  [unwired: 1 in]
        n89 = Format Value(format string="%,;%1.4f", value (0)=w65) -> (output string=w139:string)  [unwired: 1 in]
        n90 = Format Value(format string="%,;%^#_6e", value (0)=w106) -> (output string=w107:string)  [unwired: 1 in]
        n91 = Format Value(format string=" %,;%^#_6e", value (0)=w140) -> (output string=w138:string)  [unwired: 1 in]
        n92 = Format Into String(format string="[%d.4.%d.2# RESULT OF TEST RATE SCAN (V IN)]\nRATE SCAN VIN\\t%s" ("string"), initial string=w101, w77, w76, w92) -> (resulting string=w94:string)  [unwired: 1 in, 1 out]
        n93 = Build Array(w124, w123) -> (w122:string[])
        n94 = call "REPEORT.CAMBIO LINEA.vi"("Text Out"=w94) -> ("String"=w93:string)  [unwired: 8 in]
        n95 = Build Array(w122) -> (w121:string[][])
        n96 = Build Array(w139, w107, w138) -> (w135:string[])
        n97 = Build Array(w135) -> (w134:string[][])
        n98 = Format Into String(format string="%d.4.%d.3# LIMITS COMPARATION RATE SCAN" ("Secction"), w77, w76) -> (resulting string=w99:string)  [unwired: 2 in, 1 out]
        n99 = call "REPORT.Create Table.vi"("Secction"=w99, "Column Headers"=string[] ["UPPER", "LOWER"], "Text 2d"=w121, "Text In"=w93) -> ("Text Out"=w132:string)  [unwired: 4 in, 1 out]
        n100 = Format Into String(format string="%d.4.%d.4# VGA PARAMETERS RATE SCAN" ("string"), w77, w76) -> (resulting string=w96:string)  [unwired: 2 in, 1 out]
        n101 = call "REPORT.Create Table.vi"("Secction"=w96, "Column Headers"=string[] ["Amplitude (Volt)", "PULSE WIDTH (Seg)", "FRECUENCY (Hz)"], "Text 2d"=w134, "Text In"=w132) -> ("Text Out"=w133:string)  [unwired: 4 in, 1 out]
        n102 = Format Into String(format string="%d.4.%d.5# VALUES RATE SCAN ASIC (%.3g@%1.4f)" ("Secction"), w77, w76, w75, w64) -> (resulting string=w95:string)  [unwired: 2 in, 1 out]
        n103 = call "REPORT.Create Table.vi"("Secction"=w95, "Row Headers"=w78, "Column Headers"=w79, "Text 2d"=w89, "Text In"=w133) -> ("Text Out"=w74:string)  [unwired: 3 in, 1 out]
        n104 = Format Into String(format string="%d.4.%d.6# VALUES RATE SCAN ASIC RECTIFIED (%.3g@%1.4f)" ("Secction"), w77, w76, w75, w64) -> (resulting string=w91:string)  [unwired: 2 in, 1 out]
        n105 = case shown="True" TRUE {
          tunnel: w74 -> [w175 w181]
          tunnel: w91 -> [_ w180]
          tunnel: w79 -> [_ w179]
          tunnel: w78 -> [_ w178]
          tunnel: w83 -> [_ w177]
          tunnel: [w175 w176] -> w88
          frame False {
          }
          frame True {
            n106 = call "REPORT.Create Table.vi"("Secction"=w180, "Row Headers"=w178, "Column Headers"=w179, "Text 2d"=w177, "Text In"=w181) -> ("Text Out"=w176:string)  [unwired: 3 in, 1 out]
          }
        }
        n107 = call "REPEORT.CAMBIO LINEA.vi"("Text Out"=w88) -> ("String"=w105:string)  [unwired: 8 in]
      }
    }
  }
  "Text Out" <- w6
